vi "Wait For Current Play To Finish Core.vi"(9 "Timeout (seconds) (Infinity)":dbl, 11 "Sound Player in":refnum<class "Sound Player.lvclass">) -> (0 "error out":errorcluster, 3 "Sound Player out":refnum<class "Sound Player.lvclass">)   [LabVIEW 2017, in "Sound Player.lvclass"]
doc: "Wait for the sound currently playing on the player to complete. The default time out is \"Infinity\". Wiring a negative value will return an error."
uses:
  Sound Player.lvclass
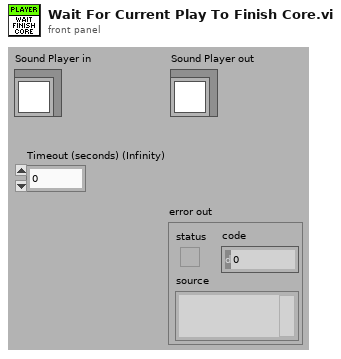
[diagram p1: front panel]
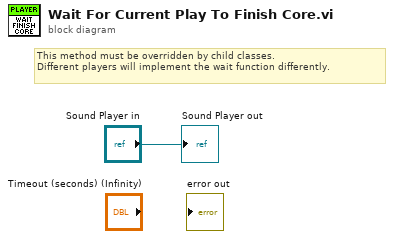
[diagram p0: block diagram]
diagram:
  # "This method must be overridden by child classes.\nDifferent players will implement the wait function differently."
  "Sound Player out" <- "Sound Player in"
